vi "PID_sctl.vi"(6 "AntiWindupInterval":fxp<+,20,4>, 7 "MeasuredValue":fxp<+/-,20,5>, 8 "Dgain":fxp<+,32,8>, 9 "Igain":fxp<+,24,10>, 10 "Pgain":fxp<+,24,8>, 11 "SetPoint":fxp<+/-,20,5>) -> (0 "Error":fxp<+/-,21,6>, 1 "ControlEffort":fxp<+/-,22,7> format="%.18g", 2 "Derivative":fxp<+/-,50,35>, 3 "RunningSum":fxp<+/-,32,8>)   [LabVIEW 2013]
uses:
  <vilib>/Platform/TimedLoop/XDataNode/timing_clust.ctl
  <vilib>/Platform/TimedLoop/XDataNode/nitl_modes.ctl
  <vilib>/Platform/TimedLoop/XDataNode/wakeup.ctl
  <vilib>/rvi/Emulation/niFpgaSctlEmulationGetInTimedLoop.vi
  <vilib>/rvi/Emulation/niFpgaEmulationReportErrorSimple.vi
  <vilib>/rvi/Emulation/niFpgaGetClockAttributes.vi
  <vilib>/rvi/Emulation/niFpgaCriticalErrorInLSC.vi
  <vilib>/Platform/TimedLoop/XDataNode/XDataNode.xnode
  <vilib>/rvi/FXPMathLib/FxpMul/XNode/nifxpmath_Multiplier.xnode
  <vilib>/rvi/FXPMathLib/FxpAdd/XNode/nifxpmath_Add.xnode
  <vilib>/rvi/FXPMathLib/FxpSub/XNode/nifxpmath_Sub.xnode
  <vilib>/Platform/TimedLoop/XDataNode/XDNodeRunTimeDep.lvlib
  <vilib>/rvi/FXPMathLib/sim/FxpSim.dll
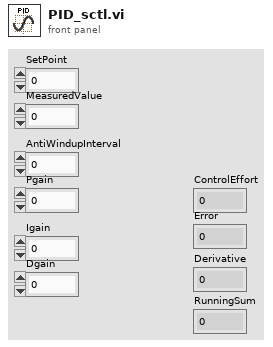
[diagram p1: front panel]
types:
  T1 = typedef "XDNodeRunTimeDep.lvlib/timing_clust.ctl" = cluster{"Expected End [f-1]":u64, "Actual End [f-1]":u64, "Finished Late? [f-1]":bool, "Expected End [i-1]":u64, "Actual End [i-1]":u64, "Finished Late? [i-1]":bool, "Expected Start [i]":u64, "Actual Start [i]":u64, "Expected Start [f]":u64, "Actual Start [f]":u64, "Source Name":string, "Structure Name":string, "Period":i64, "Deadline":i64, "Offset":i64, "Start":i64, "Priority":i32, "Timeout":i32, "Mode":T2, "Wakeup Reason":T3, "Error":errorcluster, "Source Type":string, "Secondary Source Type":string, "Global End Time":u64, "Global Start Time":u64, "Frame Duration":u64, "Iteration Duration":u64, "Assigned CPU":i32, "I/O Scan Engine Mode":u32}
  T2 = typedef "XDNodeRunTimeDep.lvlib/nitl_modes.ctl" = enum32{"No Change", "Process missed periods, maintain original phase", "Discard missed periods, maintain original phase", "Process missed periods, ignore original phase", "Discard missed periods, ignore original phase"}
  T3 = typedef "XDNodeRunTimeDep.lvlib/wakeup.ctl" = enum32{"Normal", "Aborted", "Asynchronous wakeup", "Timing source error", "Timed loop error", "Timeout"}
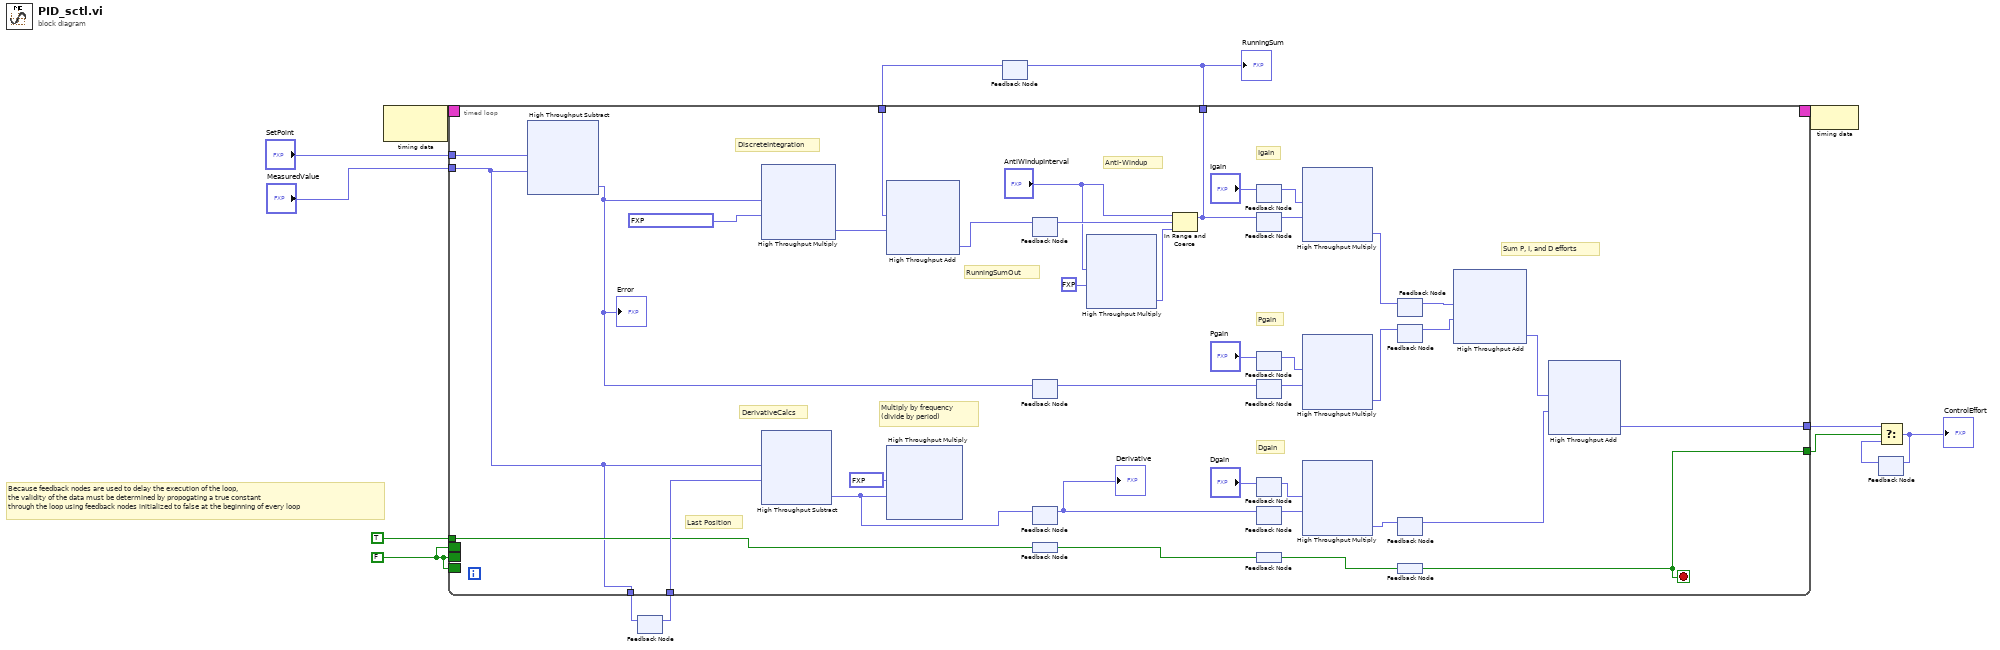
[diagram p0: block diagram]
diagram:
  w1 = FALSE
  # "Because feedback nodes are used to delay the execution of the loop, \nthe validity of the data must be determined by propogating a true constant \nthrough the loop using feedback nodes initialized to false at the beginning of every loop"
  n1 = node-c288() -> (w14:T1)  [unwired: 1 in]
  n2 = feedback #1() -> (w11:fxp<+/-,20,5>)  [unwired: 1 in]
  n3 = feedback #2() -> (w5:fxp<+/-,32,8>)  [unwired: 1 in]
  n4 = timed-loop {
    timing: w14 -> [_]
    timing-out: [_] -> w13
    tunnel: "SetPoint" -> [w24]
    tunnel: "MeasuredValue" -> [w25]
    tunnel: [w25] -> w12
    tunnel: w11 -> [w52]
    tunnel: [w15] -> w2
    tunnel: [w16] -> w7
    tunnel: TRUE -> [w34]
    border: w1 -> [_]
    border: w1 -> [_]
    tunnel: w5 -> [w31]
    tunnel: [w26] -> w4
    border: w1 -> [_]
    stop <- w16 stop-if-true
    # "Sum P, I, and D efforts"
    # "Igain"
    # "Dgain"
    # "Anti-Windup"
    # "Multiply by frequency \n(divide by period)"
    # "Last Position"
    # "RunningSumOut"
    # "Pgain"
    # "DerivativeCalcs"
    # "DiscreteIntegration"
    n5 = xnode ("High Throughput Subtract")("x"=w24, "y"=w25) -> ("x-y"=w33:fxp<+/-,21,6>)
    "Error" <- w33
    n6 = xnode ("High Throughput Multiply")("x"=w33, "y"=fxp<+,5,-13> 9.918212890625e-05) -> ("x*y"=w29:fxp<+/-,26,-7>)
    n7 = xnode "High Throughput Subtract"("x"=w25, "y"=w52) -> ("x-y"=w32:fxp<+/-,21,6>)
    n8 = xnode ("High Throughput Add")("x"=w31, "y"=w29) -> ("x+y"=w27:fxp<+/-,32,8>)
    n9 = xnode ("High Throughput Multiply")("x"=fxp<+/-,28,28> 100000.0, "y"=w32) -> ()  [unwired: 1 out]
    n10 = feedback-in #3(w27) -> ()
    n11 = feedback #3() -> (w47:fxp<+/-,32,8>)  [unwired: 1 in]
    n12 = feedback-in #4(w33) -> ()
    n13 = feedback #4() -> (w43:fxp<+/-,21,6>)  [unwired: 1 in]
    n14 = feedback-in #5(w32) -> ()
    n15 = feedback #5() -> (w42:fxp<+/-,21,6>)  [unwired: 1 in]
    "Derivative" <- w42
    n16 = feedback-in #6(w34) -> ()
    n17 = feedback #6() -> (w35:bool)
    n18 = xnode ("High Throughput Multiply")("x"="AntiWindupInterval", "y"=fxp<+/-,1,1> -1.0) -> ("x*y"=w50:fxp<+/-,21,5>)
    n19 = In Range and Coerce(upper limit="AntiWindupInterval", x=w47, lower limit=w50) -> (coerced(x)=w26:fxp<+/-,32,8>)  [unwired: 1 out]
    n20 = feedback-in #7("Igain") -> ()
    n21 = feedback #7() -> (w41:fxp<+,24,10>)  [unwired: 1 in]
    n22 = feedback-in #8(w26) -> ()
    n23 = feedback #8() -> (w46:fxp<+/-,32,8>)  [unwired: 1 in]
    n24 = feedback-in #9("Pgain") -> ()
    n25 = feedback #9() -> (w40:fxp<+,24,8>)  [unwired: 1 in]
    n26 = feedback-in #10(w43) -> ()
    n27 = feedback #10() -> (w45:fxp<+/-,21,6>)  [unwired: 1 in]
    n28 = feedback-in #11("Dgain") -> ()
    n29 = feedback #11() -> (w36:fxp<+,32,8>)  [unwired: 1 in]
    n30 = feedback-in #12(w42) -> ()
    n31 = feedback #12() -> (w44:fxp<+/-,21,6>)  [unwired: 1 in]
    n32 = feedback #13() -> (w20:bool)
    n33 = feedback-in #13(w35) -> ()
    n34 = xnode ("High Throughput Multiply")("x"=w41, "y"=w46) -> ("x*y"=w23:fxp<+/-,20,5>)
    n35 = xnode ("High Throughput Multiply")("x"=w40, "y"=w45) -> ("x*y"=w22:fxp<+/-,20,5>)
    n36 = xnode ("High Throughput Multiply")("x"=w36, "y"=w44) -> ("x*y"=w21:fxp<+/-,20,5>)
    n37 = feedback-in #14(w23) -> ()
    n38 = feedback #14() -> (w19:fxp<+/-,20,5>)  [unwired: 1 in]
    n39 = feedback-in #15(w22) -> ()
    n40 = feedback #15() -> (w18:fxp<+/-,20,5>)  [unwired: 1 in]
    n41 = feedback-in #16(w21) -> ()
    n42 = feedback #16() -> (w17:fxp<+/-,20,5>)  [unwired: 1 in]
    n43 = feedback-in #17(w20) -> ()
    n44 = feedback #17() -> (w16:bool)
    n45 = xnode ("High Throughput Add")("x"=w19, "y"=w18) -> ("x+y"=w48:fxp<+/-,21,6>)
    n46 = xnode ("High Throughput Add")("x"=w48, "y"=w17) -> ("x+y"=w15:fxp<+/-,22,7>)
  }
  "RunningSum" <- w4
  n47 = feedback-in #1(w12) -> ()
  n48 = feedback-in #2(w4) -> ()
  n49 = node-c288(w13) -> ()
  n50 = feedback #18() -> (w9:fxp<+/-,22,7>)  [unwired: 1 in]
  n51 = Select(t=w2, s=w7, f=w9) -> (s? t:f=w8:fxp<+/-,22,7>)
  "ControlEffort" <- w8
  n52 = feedback-in #18(w8) -> ()
